vi "UDP_GetDataFromDevice.vi"(5 "Remote Port":u16, 6 "timeout [ms]":i32=5000, 7 "Remote MAC Address":string, 8 "error in":errorcluster, 11 "Data":string) -> (0 "error out":errorcluster, 2 "Parameters":string[](array[string]), 3 "Command":string)   [LabVIEW 2014, in "hse-network.lvlib"]
doc: "____\nHAMPEL SOFTWARE ENGINEERING v0.7.0 (2018-07-16 18:12)"
uses:
  hse-network.lvlib
  hse-misc/Event/Event_LoadOrCreateRefs.vi
  hse-misc/hse-misc.lvlib
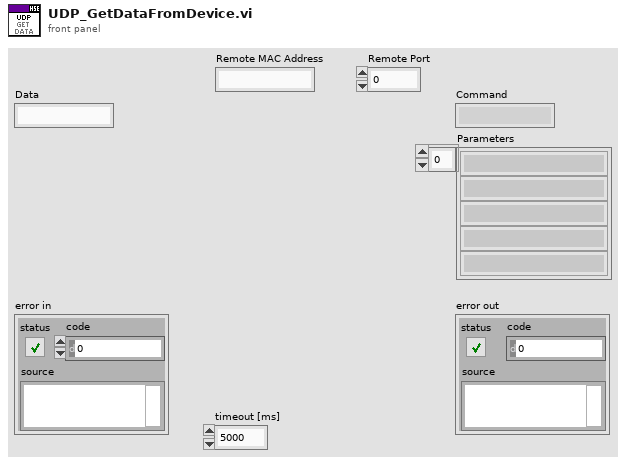
[diagram p1: front panel]
types:
  T1 = typedef "hse-misc.lvlib/Event_GenericRegistration.ctl" = refnum<event-registration>
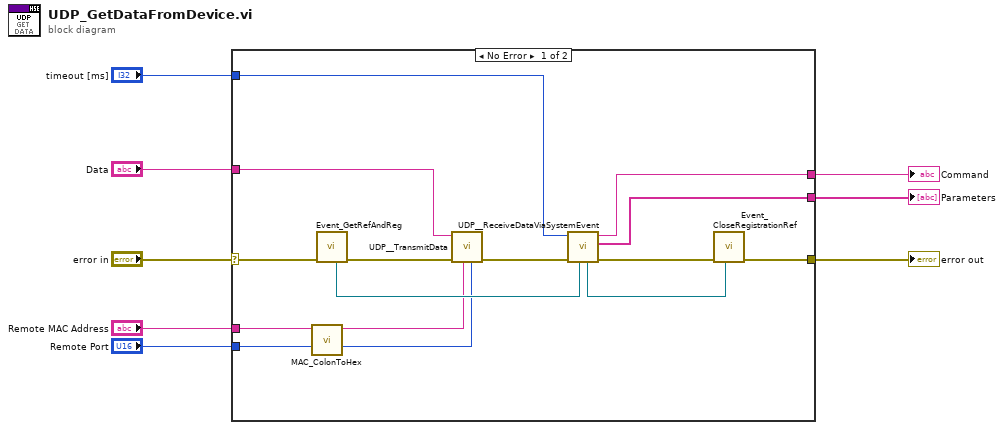
[diagram p0: block diagram]
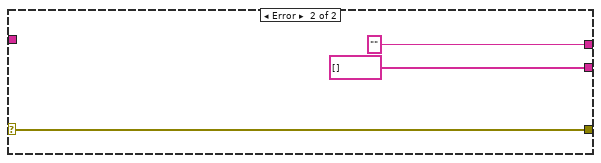
[diagram p2: hidden frame]
diagram:
  n1 = case shown="No Error" "error in" {
    selector: "error in" -> [w18 w25]
    tunnel: "Remote Port" -> [w12 _]
    tunnel: "Remote MAC Address" -> [w11 _]
    tunnel: "Data" -> [w17 _]
    tunnel: [w14 "" ("Parameter")] -> w5
    tunnel: [w19 w25] -> w4
    tunnel: "timeout [ms]" -> [w13 _]
    tunnel: [w9 string[] [] ("Parameters")] -> w1
    frame No Error {
      n2 = call "MAC_ColonToHex.vi"("MAC Address (colon notation)"=w11) -> ("MAC Address (hex string)"=w10:string)  [unwired: 10 in]
      n3 = call "Event_GetRefAndReg.vi"("error in"=w18) -> ("error out"=w22:errorcluster, "Event Registration Refnum"=w16:T1)  [unwired: 8 in, 1 out]
      n4 = call "UDP__TransmitData.vi"("Remote Port"=w12, "Remote MAC Address (hex)"=w10, "error in"=w22, "Command"=w17) -> ("error out"=w21:errorcluster)  [unwired: 7 in]
      n5 = call "UDP__ReceiveDataViaSystemEvent.vi"("Event Registration Ref IN"=w16, "error in"=w21, "Timeout"=w13) -> ("error out"=w20:errorcluster, "Parameters"=w9:string[], "Command"=w14:string, "Event Registration Ref OUT"=w15:T1)  [unwired: 5 in]
      n6 = call "Event_CloseRegistrationRef.vi"("Event Registration Refnum in"=w15, "error in (no error)"=w20) -> ("error out"=w19:errorcluster)  [unwired: 9 in]
    }
    frame Error {
    }
  }
  "error out" <- w4
  "Command" <- w5
  "Parameters" <- w1
